vi "VI_ExitApp.vi"(8 "错误输入（无错误）":errorcluster) -> (0 "错误输出":errorcluster)   [LabVIEW 2016]
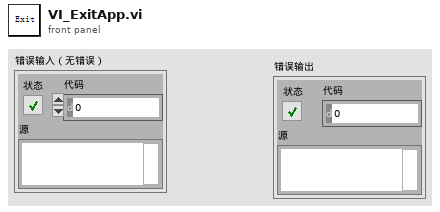
[diagram p1: front panel]
types:
  T1 = enum32{"invalid app kind", "Development System", "Run Time System", "Student Edition", "Embedded LabVIEW", "Evaluation", "Custom"}
  T2 = enum32{"Invalid", "Standard", "Closed", "Hidden", "Minimized", "Maximized"}
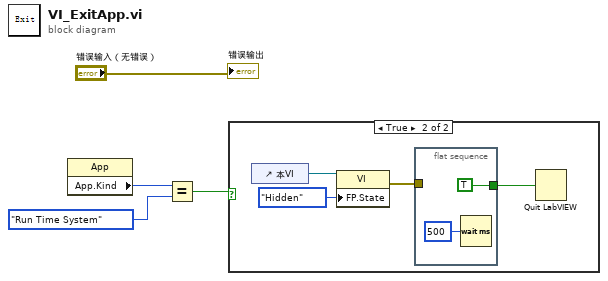
[diagram p0: block diagram]
diagram:
  n1 = property class="App"() -> ("App.Kind"=w4:T1)  [unwired: 2 in, 2 out]
  n2 = Equal?(x=w4, y=T1."Run Time System" ("应用程序:类别")) -> (x = y?=w2:bool)
  n3 = case shown="True" w2 {
    frame False {
    }
    frame True {
      n4 = control-ref of="本VI"() -> (w8:refnum<vi>)
      n5 = property class="VI"(reference=w8, "FP.State"=T2."Hidden" ("前面板窗口:状态")) -> (error out=w6:errorcluster)  [unwired: 1 in, 1 out]
      n6 = flat-sequence {
        tunnel: w6 -> [_]
        tunnel: [TRUE] -> w5
        frame #0 {
          n7 = Wait (ms)(milliseconds to wait=u32 500 ("等待时间（毫秒）")) -> ()  [unwired: 1 out]
        }
      }
      n8 = Quit LabVIEW(quit? (T)=w5) -> ()
    }
  }
  "错误输出" <- "错误输入（无错误）"
